vi "Scripting_FollowWireLeft.vi"(0 "Term Refnum":refnum<vi>, 2 "NodeTypesToFind":string[](array[string]), 3 "CreateParentTerminals(False)":bool, 5 "error in":errorcluster, 6 "MainitainDataType":bool, 7 "StopCriteria":T1) -> (15 "Nodes":refnum<vi>[](array[refnum]), 16 "NodeTypes":string[](array[string]), 17 "ParentTerminal":refnum<vi>[](array[refnum]), 19 "error out":errorcluster)   [LabVIEW 2016]
uses:
  <resource>/Framework/Providers/Open_GDS/ClassProviders/Common/ScriptingFunctions/Scripting_FollowWireDownStreams_StopCriteria.ctl
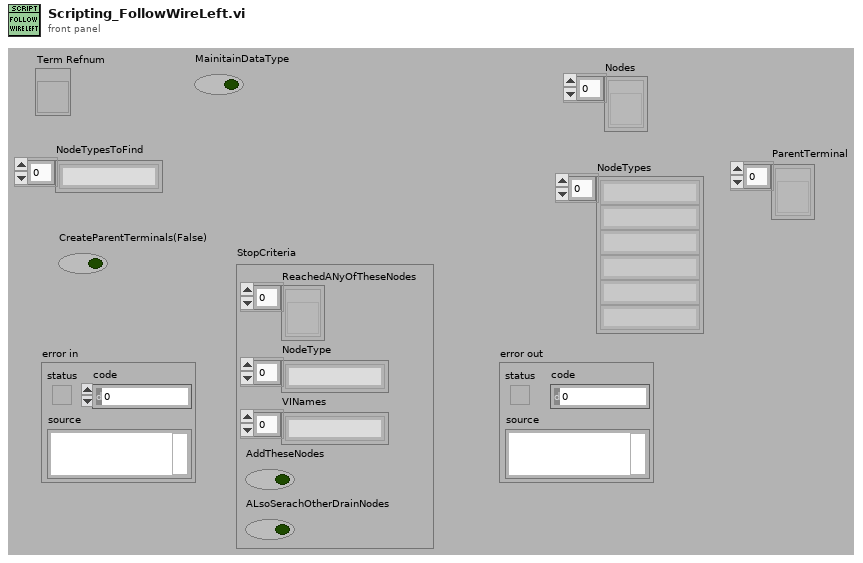
[diagram p1: front panel]
types:
  T1 = typedef "Scripting_FollowWireDownStreams_StopCriteria.ctl" = cluster{"ReachedANyOfTheseNodes":refnum<vi>[], "NodeType":string[], "VINames":string[], "AddTheseNodes":bool, "ALsoSerachOtherDrainNodes":bool}
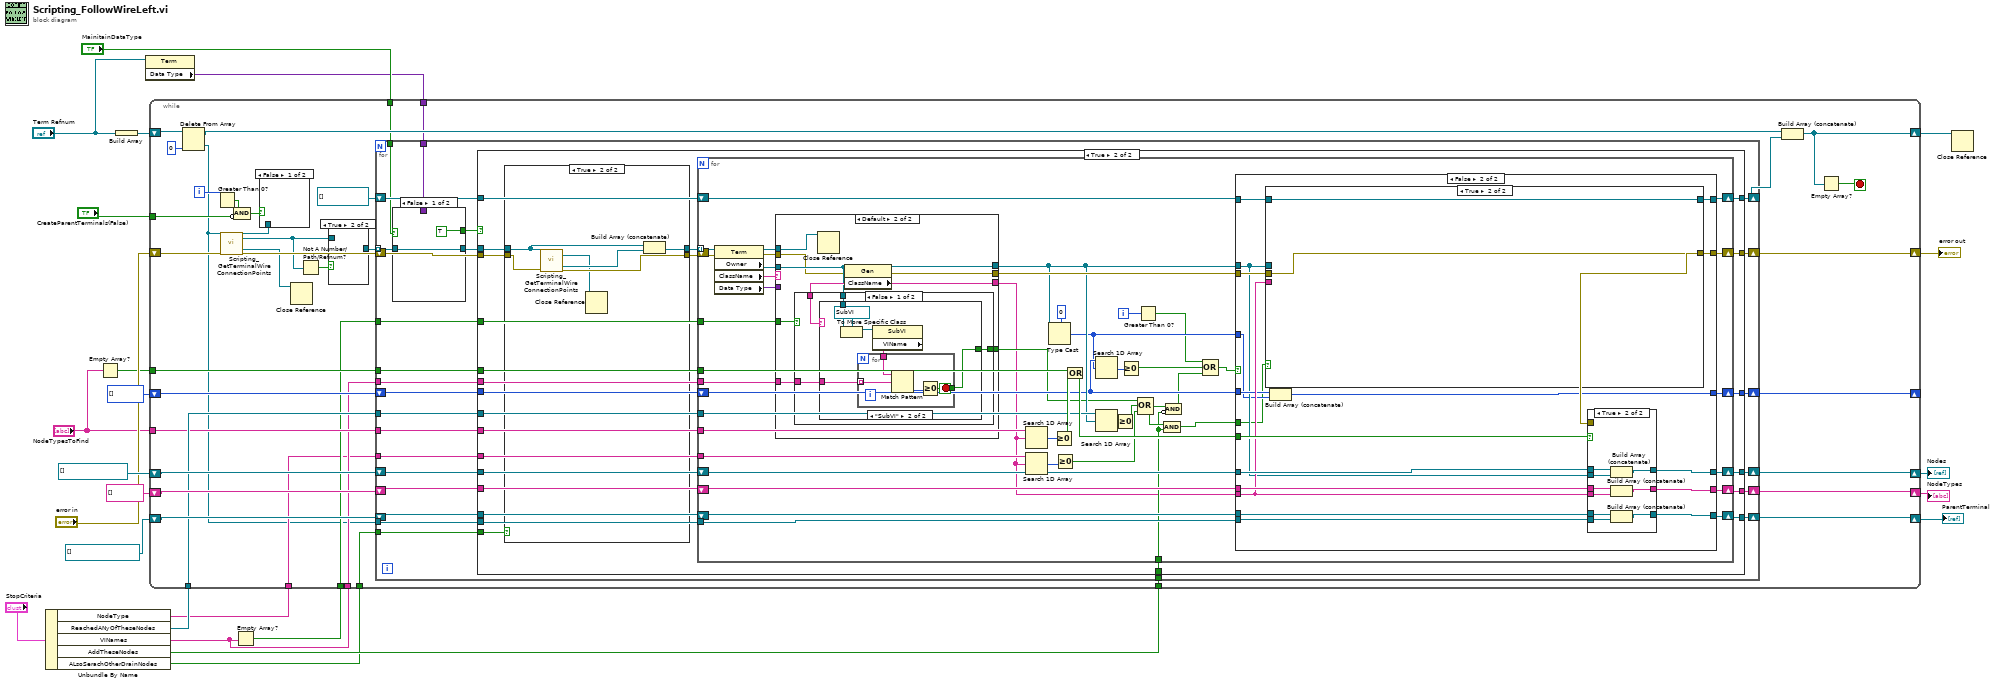
[diagram p0: block diagram]
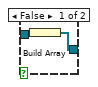
[diagram p2: hidden frame]
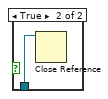
[diagram p3: hidden frame]
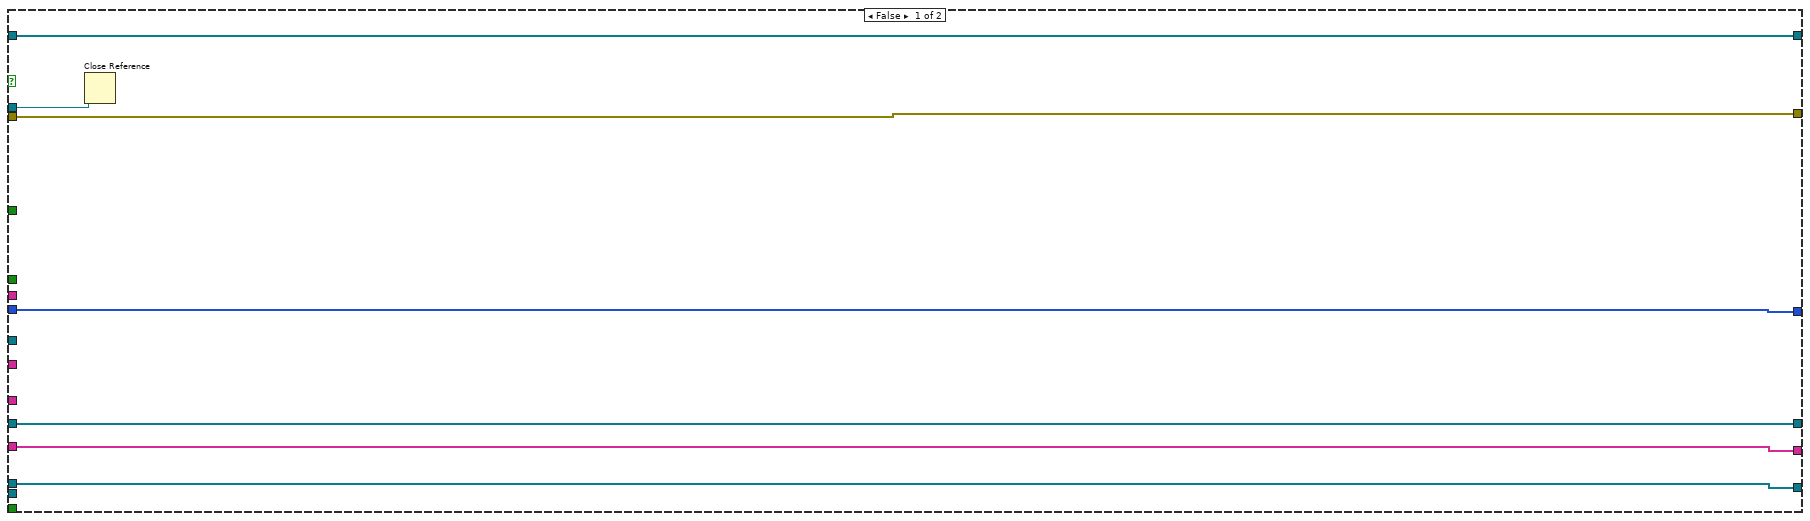
[diagram p4: hidden frame]
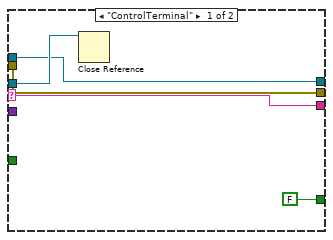
[diagram p5: hidden frame]
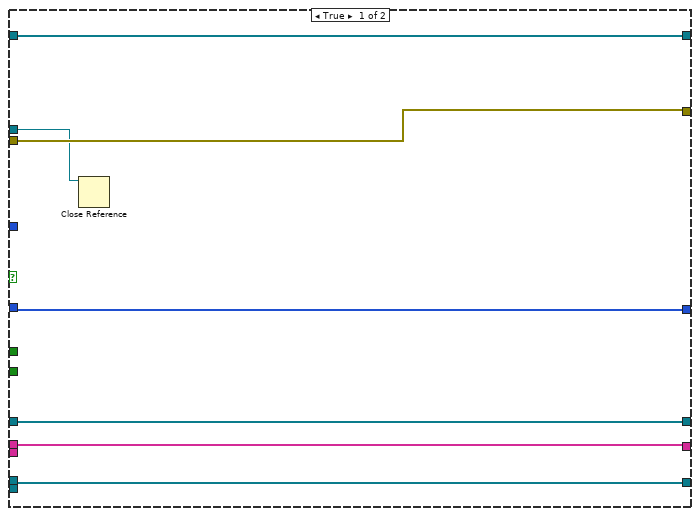
[diagram p8: hidden frame]
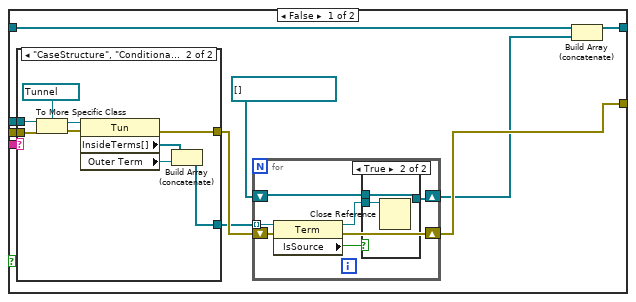
[diagram p9: hidden frame]
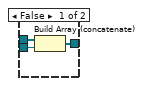
[diagram p10: hidden frame]
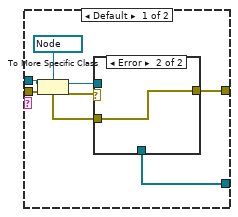
[diagram p11: hidden frame]
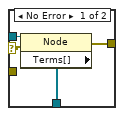
[diagram p12: hidden frame]
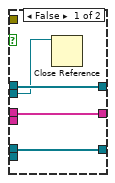
[diagram p13: hidden frame]
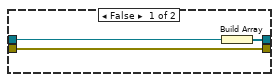
[diagram p14: hidden frame]
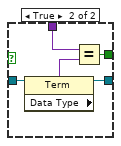
[diagram p15: hidden frame]
diagram:
  n1 = Unbundle By Name("StopCriteria") -> ("NodeType"=w5:string[], "ReachedANyOfTheseNodes"=w12:refnum<vi>[], "VINames"=w7:string[], "AddTheseNodes"=w6:bool, "ALsoSerachOtherDrainNodes"=w1:bool)
  n2 = Empty Array?(array="NodeTypesToFind") -> (empty?=w9:bool)
  n3 = Build Array("Term Refnum") -> (w23:refnum<vi>[])
  n4 = property class="Term"(reference="Term Refnum") -> ("Data Type"=w2:variant)  [unwired: 1 in, 2 out]
  n5 = Empty Array?(array=w7) -> (empty?=w8:bool)
  n6 = while {
    shift-right: [w53] -> w24
    shift-left: w23 -> [w62]
    tunnel: "NodeTypesToFind" -> [w41]
    shift-right: [w56] -> w19
    shift-left: refnum<vi>[] [] -> [w57]
    shift-right: [w55] -> w21
    shift-left: "error in" -> [w54]
    shift-right: [w50] -> w17
    shift-left: string[] [] -> [w49]
    shift-right: [w47] -> w16
    shift-left: refnum<vi>[] [] ("ParentTerminal") -> [w48]
    tunnel: "CreateParentTerminals(False)" -> [w44]
    tunnel: w12 -> [w42]
    shift-right: [w39] -> _
    shift-left: u32[] [] -> [w40]
    tunnel: w9 -> [w37]
    tunnel: w8 -> [w36]
    tunnel: w7 -> [w35]
    tunnel: w6 -> [w34]
    tunnel: w5 -> [w29]
    tunnel: "MainitainDataType" -> [w28]
    tunnel: w2 -> [w27]
    tunnel: w1 -> [w25]
    i -> [w46]
    stop <- w52 stop-if-true
    n7 = Delete From Array(array=w62, index=0) -> (deleted portion=w26:refnum<vi>, array with subset deleted=w61:refnum<vi>[])  [unwired: 1 in]
    n8 = Greater Than 0?(x=w46) -> (x > 0?=w45:bool)
    n9 = call <resource>:"Scripting_GetTerminalWireConnectionPoints.vi"("Term Refnum In"=w26, "error in"=w54) -> ("Term Refnum Out"=w51:refnum<vi>, "WireTermSource"=w31:refnum<vi>, "AllWireTerminalDrains"=w33:refnum<vi>[], "error out"=w59:errorcluster)  [unwired: 9 in, 5 out]
    n10 = Compound Arithmetic op=AND(w45, invert w44) -> (w43:bool)
    n11 = case shown="False" w43 {
      tunnel: w51 -> [_ w65]
      frame False {
      }
      frame True {
        n12 = Close Reference(reference=w65) -> ()  [unwired: 1 in, 1 out]
      }
    }
    n13 = Close Reference(reference=w33) -> ()  [unwired: 1 in, 1 out]
    n14 = Not A Number/Path/Refnum?(number/path/refnum=w31) -> (NaN/Path/Refnum?=w30:bool)
    n15 = case shown="True" w30 {
      tunnel: [w64 _] -> w32
      tunnel: w31 -> [w63 _]
      frame False {
        n16 = Build Array(w63) -> (w64:refnum<vi>[])
      }
      frame True {
      }
    }
    n17 = for {
      tunnel: w32 -> [w71] mode=indexing
      tunnel: w41 -> [w80]
      shift-right: [w90] -> w56
      shift-left: w57 -> [w91]
      shift-right: [w84] -> w55
      shift-left: w59 -> [w89]
      shift-right: [w88] -> w58
      shift-left: refnum<vi>[] [] -> [w87]
      shift-right: [w86] -> w50
      shift-left: w49 -> [w85]
      shift-right: [w82] -> w47
      shift-left: w48 -> [w83]
      tunnel: w26 -> [w81]
      tunnel: w42 -> [w78]
      tunnel: w37 -> [w79]
      shift-right: [w77] -> w39
      shift-left: w40 -> [w76]
      tunnel: w36 -> [w75]
      tunnel: w35 -> [w74]
      tunnel: w34 -> [w73]
      tunnel: w29 -> [w72]
      tunnel: w28 -> [w69]
      tunnel: w27 -> [w68]
      tunnel: w25 -> [w66]
      n18 = case shown="False" w69 {
        tunnel: w71 -> [w291 w296]
        tunnel: [w291 w295] -> w70
        tunnel: w68 -> [_ w293]
        tunnel: [TRUE w292] -> w67
        frame False {
        }
        frame True {
          n19 = property class="Term"(reference=w296) -> (reference out=w295:refnum<vi>, "Data Type"=w294:variant)  [unwired: 1 in, 1 out]
          n20 = Equal?(x=w293, y=w294) -> (x = y?=w292:bool)
        }
      }
      n21 = case shown="True" w67 {
        tunnel: w91 -> [w94 w122]
        tunnel: [w94 w121] -> w90
        tunnel: w89 -> [w96 w102]
        tunnel: [w97 w120] -> w88
        tunnel: w87 -> [w97 w101]
        tunnel: [w93 w119] -> w86
        tunnel: w85 -> [w93 w118]
        tunnel: [w96 w117] -> w84
        tunnel: w83 -> [w92 w116]
        tunnel: [w92 w115] -> w82
        tunnel: w81 -> [_ w114]
        tunnel: w80 -> [_ w113]
        tunnel: w79 -> [_ w112]
        tunnel: w78 -> [_ w111]
        tunnel: [w95 w110] -> w77
        tunnel: w76 -> [w95 w109]
        tunnel: w75 -> [_ w108]
        tunnel: w74 -> [_ w107]
        tunnel: w73 -> [_ w106]
        tunnel: w72 -> [_ w105]
        tunnel: w70 -> [w98 w103]
        tunnel: w66 -> [_ w104]
        frame False {
          n22 = Close Reference(reference=w98) -> ()  [unwired: 1 in, 1 out]
        }
        frame True {
          n23 = case shown="True" w104 {
            tunnel: w103 -> [w282 w287]
            tunnel: w102 -> [w281 w289]
            tunnel: [w283 w285] -> w100
            tunnel: [w281 w288] -> w99
            frame False {
              n24 = Build Array(w282) -> (w283:refnum<vi>[])
            }
            frame True {
              n25 = call <resource>:"Scripting_GetTerminalWireConnectionPoints.vi"("Term Refnum In"=w287, "error in"=w289) -> ("WireTermSource"=w284:refnum<vi>, "AllWireTerminalDrains"=w286:refnum<vi>[], "error out"=w288:errorcluster)  [unwired: 9 in, 6 out]
              n26 = Close Reference(reference=w284) -> ()  [unwired: 1 in, 1 out]
              n27 = Build Array (concatenate)(w287, w286) -> (w285:refnum<vi>[])
            }
          }
          n28 = for {
            tunnel: w114 -> [w159]
            tunnel: w113 -> [w158]
            tunnel: w112 -> [w157]
            tunnel: w111 -> [w154]
            tunnel: w108 -> [w144]
            tunnel: w107 -> [w142]
            tunnel: w106 -> [w137]
            tunnel: w105 -> [w132]
            tunnel: w100 -> [w127] mode=indexing
            shift-right: [w167] -> w120
            shift-left: w101 -> [w126]
            shift-right: [w153] -> w110
            shift-left: w109 -> [w150]
            shift-right: [w160] -> w115
            shift-left: w116 -> [w161]
            shift-right: [w165] -> w119
            shift-left: w118 -> [w164]
            shift-right: [w168] -> w121
            shift-left: w122 -> [w169]
            shift-right: [w162] -> w117
            shift-left: w99 -> [w123]
            i -> [w125]
            n29 = property class="Term"(reference=w127, error in=w123) -> (reference out=w133:refnum<vi>, error out=w135:errorcluster, "Owner"=w143:refnum<vi>, "ClassName"=w134:string, "Data Type"=w128:variant)
            n30 = case shown="Default" w134 {
              selector: w134 -> [w174 _]
              tunnel: [w173 w183] -> w163
              tunnel: [w171 w182] -> w152
              tunnel: w144 -> [_ w181]
              tunnel: [w174 w180] -> w131
              tunnel: w143 -> [w172 w179]
              tunnel: w142 -> [_ w178]
              tunnel: [FALSE w177] -> w140
              tunnel: w135 -> [w173 w176]
              tunnel: w133 -> [w171 w175]
              tunnel: w128 -> [_ _]
              frame "ControlTerminal" {
                n31 = Close Reference(reference=w172) -> ()  [unwired: 1 in, 1 out]
              }
              frame Default {
                n32 = Close Reference(reference=w175) -> ()  [unwired: 1 in, 1 out]
                n33 = property class="Gen"(reference=w179, error in=w176) -> (reference out=w182:refnum<vi>, error out=w183:errorcluster, "ClassName"=w180:string)
                n34 = case shown="False" w181 {
                  tunnel: w180 -> [w187 _]
                  tunnel: w179 -> [w186 _]
                  tunnel: w178 -> [w185 _]
                  tunnel: [w184 _] -> w177
                  frame False {
                    n35 = case shown="\"SubVI\"" w187 {
                      tunnel: w186 -> [_ w193]
                      tunnel: w185 -> [_ w189]
                      tunnel: [_ w188] -> w184
                      frame Default {
                      }
                      frame "SubVI" {
                        n36 = To More Specific Class(target class=refnum<vi> refnum ("Owner"), reference=w193) -> (specific class reference=w191:refnum<vi>)  [unwired: 1 in, 1 out]
                        n37 = property class="SubVI"(reference=w191) -> ("VIName"=w190:string)  [unwired: 1 in, 2 out]
                        n38 = for {
                          tunnel: w190 -> [w197]
                          tunnel: w189 -> [w196] mode=indexing
                          tunnel: [w194] -> w188
                          stop <- w194 stop-if-true
                          n39 = Match Pattern(string=w197, regular expression=w196) -> (offset past match=w195:i32)  [unwired: 1 in, 3 out]
                          n40 = Greater Or Equal To 0?(x=w195) -> (x >= 0?=w194:bool)
                        }
                      }
                    }
                  }
                  frame True {
                  }
                }
              }
            }
            n41 = Search 1D Array(1D array=w158, element=w131) -> (index of element=w166:i32)  [unwired: 1 in]
            n42 = Search 1D Array(1D array=w132, element=w131) -> (index of element=w130:i32)  [unwired: 1 in]
            n43 = Type Cast(type=u32 0 ("index"), x=w152) -> (*(type *) &x=w149:u32)
            n44 = Greater Or Equal To 0?(x=w166) -> (x >= 0?=w156:bool)
            n45 = Greater Or Equal To 0?(x=w130) -> (x >= 0?=w129:bool)
            n46 = Or(x=w157, y=w156) -> (x .or. y?=w155:bool)
            n47 = Search 1D Array(1D array=w150, element=w149) -> (index of element=w147:i32)  [unwired: 1 in]
            n48 = Search 1D Array(1D array=w154, element=w152) -> (index of element=w148:i32)  [unwired: 1 in]
            n49 = Greater Or Equal To 0?(x=w148) -> (x >= 0?=w141:bool)
            n50 = Greater Or Equal To 0?(x=w147) -> (x >= 0?=w146:bool)
            n51 = Greater Than 0?(x=w125) -> (x > 0?=w124:bool)
            n52 = Compound Arithmetic op=OR(w140, w141, w129) -> (w138:bool)
            n53 = Compound Arithmetic op=AND(w138, w137) -> (w136:bool)
            n54 = Compound Arithmetic op=AND(w138, invert w137) -> (w139:bool)
            n55 = Compound Arithmetic op=OR(w124, w146, w139) -> (w145:bool)
            n56 = case shown="False" w145 {
              tunnel: w169 -> [w202 w222]
              tunnel: [w202 w221] -> w168
              tunnel: [w204 w220] -> w167
              tunnel: w126 -> [w204 w219]
              tunnel: w155 -> [_ w218]
              tunnel: [w201 w217] -> w165
              tunnel: w164 -> [w201 w216]
              tunnel: w163 -> [w203 w215]
              tunnel: w131 -> [_ w214]
              tunnel: [w203 w210] -> w162
              tunnel: w161 -> [w200 w213]
              tunnel: [w200 w212] -> w160
              tunnel: w159 -> [_ w211]
              tunnel: w152 -> [w199 w208]
              tunnel: w150 -> [w198 w209]
              tunnel: [w198 w207] -> w153
              tunnel: w149 -> [_ w206]
              tunnel: w136 -> [_ w205]
              frame True {
                n57 = Close Reference(reference=w199) -> ()  [unwired: 1 in, 1 out]
              }
              frame False {
                n58 = case shown="True" w205 {
                  tunnel: [w232 w266] -> w220
                  tunnel: w219 -> [w231 w266]
                  tunnel: w215 -> [w230 w267]
                  tunnel: w214 -> [w229 _]
                  tunnel: [w226 w267] -> w210
                  tunnel: w208 -> [w224 _]
                  frame False {
                    n59 = case shown="\"CaseStructure\", \"ConditionalTunnel\", \"LeftShiftRegister\", \"LoopTunnel\", \"RightShiftRegister\", \"SelectorTunnel\", \"Tunnel\"" w229 {
                      tunnel: w230 -> [w245 w264]
                      tunnel: [w248 w261] -> w228
                      tunnel: w224 -> [w249 w260]
                      tunnel: [w247 w257] -> w227
                      frame Default {
                        n60 = To More Specific Class(target class=refnum<vi> refnum ("Owner"), reference=w249, error in=w245) -> (specific class reference=w250:refnum<vi>, error out=w246:errorcluster)
                        n61 = case shown="Error" w246 {
                          selector: w246 -> [w252 _]
                          tunnel: w250 -> [w255 _]
                          tunnel: [w254 w256] -> w248
                          tunnel: [w253 _] -> w247
                          tunnel: w245 -> [_ w256]
                          frame No Error {
                            n62 = property class="Node"(reference=w255, error in=w252) -> (error out=w254:errorcluster, "Terms[]"=w253:refnum<vi>[])  [unwired: 1 out]
                          }
                          frame Error {
                          }
                        }
                      }
                      frame "CaseStructure", "ConditionalTunnel", "LeftShiftRegister", "LoopTunnel", "RightShiftRegister", "SelectorTunnel", "Tunnel" {
                        n63 = To More Specific Class(target class=refnum<vi> refnum ("reference"), reference=w260, error in=w264) -> (specific class reference=w263:refnum<vi>, error out=w262:errorcluster)
                        n64 = property class="Tun"(reference=w263, error in=w262) -> (error out=w261:errorcluster, "InsideTerms[]"=w259:refnum<vi>[], "Outer Term"=w258:refnum<vi>)  [unwired: 1 out]
                        n65 = Build Array (concatenate)(w259, w258) -> (w257:refnum<vi>[])
                      }
                    }
                    n66 = for {
                      tunnel: w227 -> [w239] mode=indexing
                      shift-right: [w237] -> w226
                      shift-left: w228 -> [w238]
                      shift-right: [w233] -> w225
                      shift-left: refnum<vi>[] [] -> [w236]
                      n67 = property class="Term"(reference=w239, error in=w238) -> (reference out=w234:refnum<vi>, error out=w237:errorcluster, "IsSource"=w235:bool)
                      n68 = case shown="True" w235 {
                        tunnel: w236 -> [w242 w244]
                        tunnel: w234 -> [w241 w243]
                        tunnel: [w240 w244] -> w233
                        frame False {
                          n69 = Build Array (concatenate)(w242, w241) -> (w240:refnum<vi>[])
                        }
                        frame True {
                          n70 = Close Reference(reference=w243) -> ()  [unwired: 1 in, 1 out]
                        }
                      }
                    }
                    n71 = Build Array (concatenate)(w231, w225) -> (w232:refnum<vi>[])
                  }
                  frame True {
                  }
                }
                n72 = Build Array (concatenate)(w209, w206) -> (w207:u32[])
                n73 = case shown="True" w218 {
                  tunnel: w222 -> [w271 w280]
                  tunnel: [w271 w279] -> w221
                  tunnel: w214 -> [_ w276]
                  tunnel: w216 -> [w270 w277]
                  tunnel: [w270 w278] -> w217
                  tunnel: w208 -> [w269 w275]
                  tunnel: w210 -> [_ _]
                  tunnel: w211 -> [_ w274]
                  tunnel: w213 -> [w268 w273]
                  tunnel: [w268 w272] -> w212
                  frame False {
                    n74 = Close Reference(reference=w269) -> ()  [unwired: 1 in, 1 out]
                  }
                  frame True {
                    n75 = Build Array (concatenate)(w280, w275) -> (w279:refnum<vi>[])
                    n76 = Build Array (concatenate)(w277, w276) -> (w278:string[])
                    n77 = Build Array (concatenate)(w273, w274) -> (w272:refnum<vi>[])
                  }
                }
              }
            }
          }
        }
      }
    }
    n78 = Build Array (concatenate)(w61, w58) -> (w53:refnum<vi>[])
    n79 = Empty Array?(array=w53) -> (empty?=w52:bool)
  }
  "error out" <- w21
  "Nodes" <- w19
  "NodeTypes" <- w17
  "ParentTerminal" <- w16
  n80 = Close Reference(reference=w24) -> ()  [unwired: 1 in, 1 out]
